vi "Word Game Solution.vi"() -> ()   [LabVIEW 2015]
uses:
  TypeDef/Word Statistic.ctl
  TypeDef/Word.ctl
panel:
  in  "Word 6":T1
  in  "Word 5":T1
  in  "Word 4":T1
  in  "Word 3":T1
  in  "Word 2":T1
  in  "Word 1":T1
  in  "Reset":bool
  out "Word Statistic Any":T2[](array[typedef])
  out "Count":i32
  out "Word Statistic Letter":T2[](array[typedef])
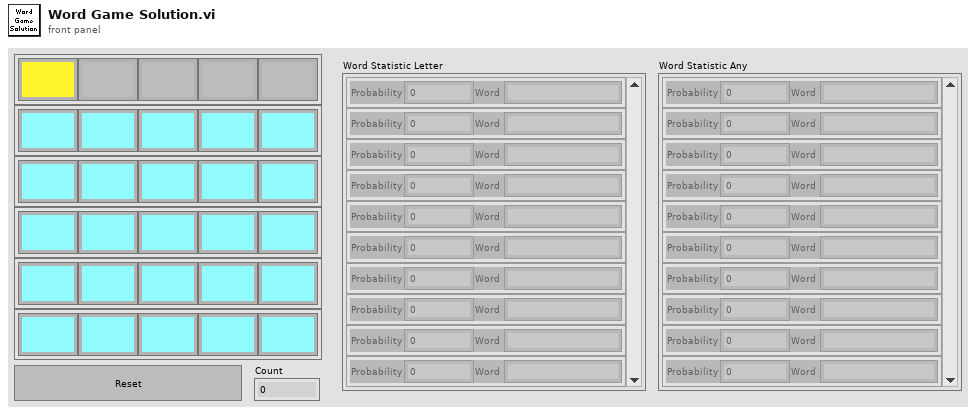
[diagram p1: front panel]
types:
  T1 = typedef "Word.ctl" = cluster{"1":string, "2":string, "3":string, "4":string, "5":string}
  T2 = typedef "Word Statistic.ctl" = cluster{"Probability":dbl, "Word":string}
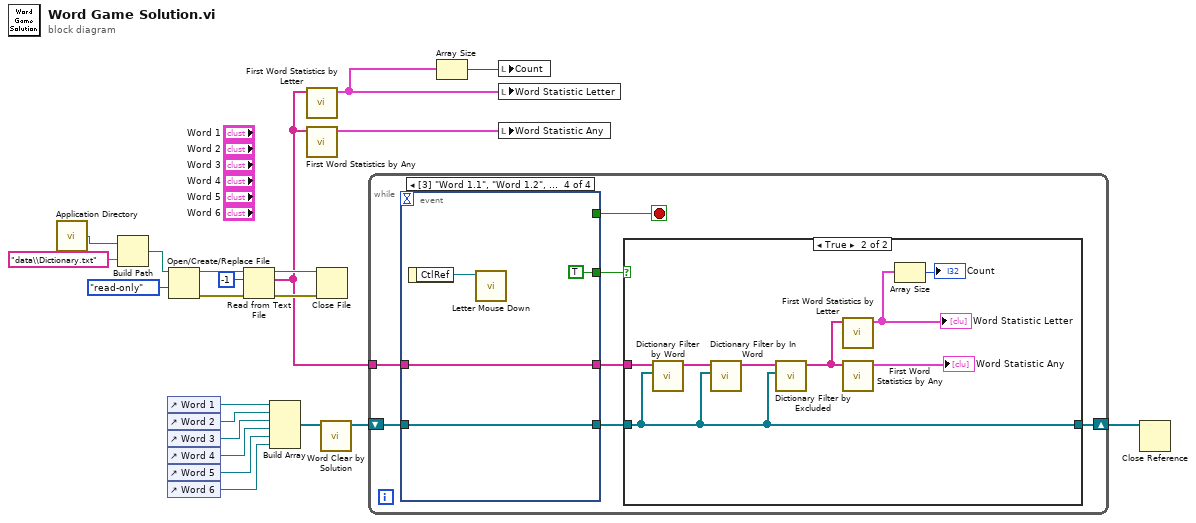
[diagram p0: block diagram]
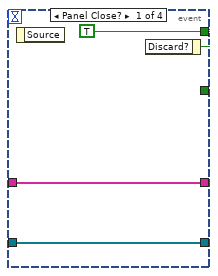
[diagram p3: hidden frame]
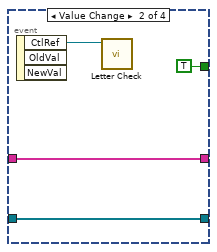
[diagram p4: hidden frame]
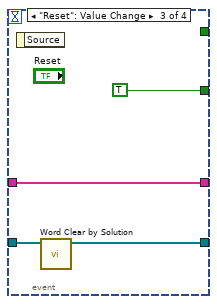
[diagram p5: hidden frame]
diagram:
  n1 = call <vilib>:"Application Directory.vi"() -> ("Application Directory"=w14:path)
  n2 = Build Path(base path=w14, name or relative path="data\\Dictionary.txt") -> (appended path=w16:path)
  n3 = control-ref of="Word 1"() -> (w9:refnum<vi>)
  n4 = control-ref of="Word 2"() -> (w8:refnum<vi>)
  n5 = control-ref of="Word 3"() -> (w7:refnum<vi>)
  n6 = control-ref of="Word 4"() -> (w6:refnum<vi>)
  n7 = control-ref of="Word 5"() -> (w5:refnum<vi>)
  n8 = control-ref of="Word 6"() -> (w4:refnum<vi>)
  n9 = Open/Create/Replace File(file path (use dialog)=w16, access (0:read/write)=enum16{"read/write", "read-only", "write-only"}."read-only") -> (refnum out=w21:refnum<file>, error out=w20:errorcluster)  [unwired: 4 in, 1 out]
  n10 = Read from Text File(file (use dialog)=w21, count=-1, error in=w20) -> (refnum out=w18:refnum<file>, text=w11:string[], error out=w17:errorcluster)  [unwired: 1 in, 1 out]
  n11 = Build Array(w9, w8, w7, w6, w5, w4) -> (w3:refnum<vi>[])
  n12 = call "First Word Statistics by Letter.vi"("Dictionary"=w11) -> ("Word Statistic"=w12:T2[])  [unwired: 10 in]
  n13 = call "First Word Statistics by Any.vi"("Dictionary"=w11) -> ("Word Statistic"=w10:T2[])  [unwired: 10 in]
  n14 = Close File(refnum=w18, error in=w17) -> ()  [unwired: 2 out]
  n15 = call "Word Clear by Solution.vi"("Words_Ref in"=w3) -> ("Words_Ref out"=w2:refnum<vi>[])  [unwired: 10 in]
  n16 = while {
    tunnel: w11 -> [w28]
    shift-right: [w24] -> w1
    shift-left: w2 -> [w26]
    stop <- w29 stop-if-true
    n17 = event shown="[3] \"Word 1.1\", \"Word 1.2\", \"Word 1.3\", \"Word 1.4\", \"Word 1.5\", \"Word 2.1\", \"Word 2.2\", \"Word 2.3\", \"Word 2.4\", \"Word 2.5\", \"Word 3.1\", \"Word 3.2\", \"Word 3.3\", \"Word 3.4\", \"Word 3.5\", \"Word 4.1\", \"Word 4.2\", \"Word 4.3\", \"Word 4.4\", \"Word 4.5\", \"Word 5.1\", \"Word 5.2\", \"Word 5.3\", \"Word 5.4\", \"Word 5.5\", \"Word 6.1\", \"Word 6.2\", \"Word 6.3\", \"Word 6.4\", \"Word 6.5\": Mouse Down" {
      selector: _ -> [_ _ _ _]
      dyn-events: _ -> [_ _ _ _]
      timeout: _ -> [_ _ _ _]
      tunnel: [w41 _ _ _] -> w29
      tunnel: w28 -> [w40 w45 w49 w53]
      tunnel: [w40 w45 w49 w53] -> w27
      tunnel: w26 -> [w39 w43 w48 w52]
      tunnel: [w39 w43 w47 w52] -> w25
      tunnel: [_ TRUE TRUE TRUE] -> w23
      event Panel Close? {
        w41 = TRUE
        n18 = event-data() -> ()  [unwired: 1 in, 1 out]
        n19 = event-data("Discard?"=w41) -> ()  [unwired: 1 in, 1 out]
      }
      event Value Change {
        n20 = event-data() -> ("CtlRef"=w44:refnum<vi>)  [unwired: 1 in, 2 out]
        n21 = call "Letter Check.vi"("Letter_Ref"=w44) -> ()  [unwired: 11 in]
      }
      event "Reset": Value Change {
        n22 = event-data() -> ()  [unwired: 1 in, 1 out]
        n23 = call "Word Clear by Solution.vi"("Words_Ref in"=w48) -> ("Words_Ref out"=w47:refnum<vi>[])  [unwired: 10 in]
      }
      event Mouse Down {
        n24 = event-data() -> ("CtlRef"=w51:refnum<vi>)  [unwired: 1 in]
        n25 = call "Letter Mouse Down.vi"("Letter_Ref"=w51) -> ()  [unwired: 11 in]
      }
    }
    n26 = case shown="True" w23 {
      tunnel: w27 -> [_ w38]
      tunnel: w25 -> [w30 w31]
      tunnel: [w30 w31] -> w24
      frame False {
      }
      frame True {
        n27 = call "Dictionary Filter by Word.vi"("Words_Ref in"=w31, "Dictionary in"=w38) -> ("Dictionary out"=w33:string[])  [unwired: 9 in]
        n28 = call "Dictionary Filter by In Word.vi"("Words_Ref in"=w31, "Dictionary in"=w33) -> ("Dictionary out"=w32:string[])  [unwired: 9 in]
        n29 = call "Dictionary Filter by Excluded.vi"("Words_Ref in"=w31, "Dictionary in"=w32) -> ("Dictionary out"=w35:string[])  [unwired: 9 in]
        n30 = call "First Word Statistics by Letter.vi"("Dictionary"=w35) -> ("Word Statistic"=w37:T2[])  [unwired: 10 in]
        "Word Statistic Letter" <- w37
        n31 = call "First Word Statistics by Any.vi"("Dictionary"=w35) -> ("Word Statistic"=→"Word Statistic Any":T2[])  [unwired: 10 in]
        n32 = Array Size(array=w37) -> (size(s)=→"Count":i32)
      }
    }
  }
  n33 = Array Size(array=w12) -> (size(s)=w13:i32)
  n34 = local write "Count"(w13) -> ()
  n35 = local write "Word Statistic Letter"(w12) -> ()
  n36 = local write "Word Statistic Any"(w10) -> ()
  n37 = Close Reference(reference=w1) -> ()  [unwired: 1 in, 1 out]
